vi "Write Time Remaining.vi"(8 "error in (no error)":errorcluster, 11 "Value":dbl) -> (0 "error out":errorcluster)   [LabVIEW 2015, in "UI Handler.lvclass"]
uses:
  UI Handler.lvclass
  UI Handler.lvclass/UI Handler.ctl
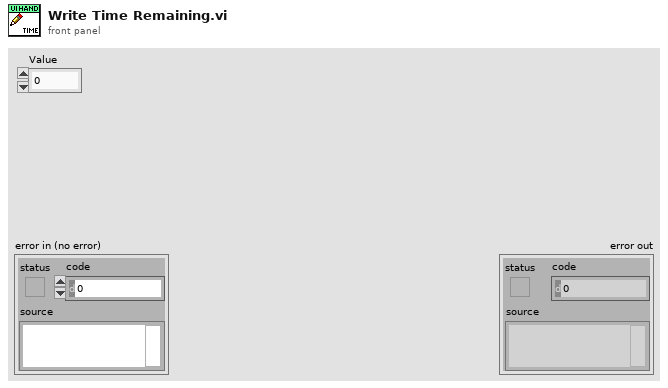
[diagram p1: front panel]
types:
  T1 = typedef "UI Handler.lvclass/Session Handle.ctl" = refnum<data-value>
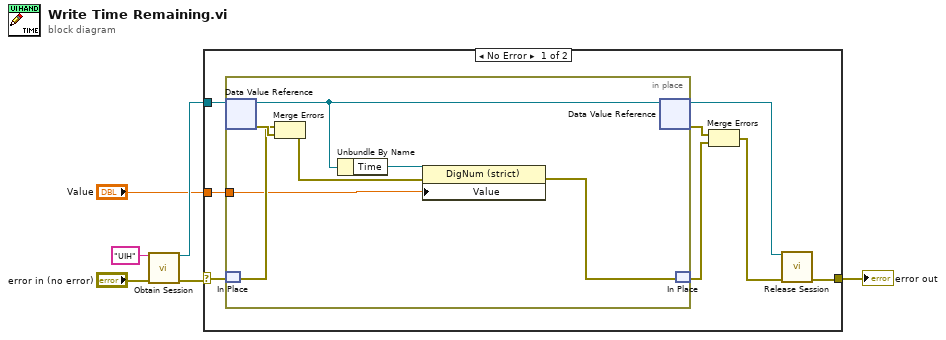
[diagram p0: block diagram]
diagram:
  n1 = call "Obtain Session.vi"("Session  Name ()"="UIH", "error in (no error)"="error in (no error)") -> ("Session Handle"=w2:T1, "error out"=w3:errorcluster)  [unwired: 12 in]
  n2 = case shown="No Error" w3 {
    selector: w3 -> [w11 w22]
    tunnel: w2 -> [w14 _]
    tunnel: [w7 w22] -> w5
    tunnel: "Value" -> [w10 _]
    frame No Error {
      n3 = in-place {
        in-place-border: w10 -> [w15]
        n4 = in-place-dvr #1(w14) -> (w19:refnum<class "UI Handler.lvclass">, w21:errorcluster)
        n5 = in-place-match #2(w11) -> (w20:errorcluster)
        n6 = Merge Errors(w20, w21) -> (w17:errorcluster)
        n7 = Unbundle By Name(w19) -> ("Time"=w18:refnum<vi>)
        n8 = property class="DigNum (strict)"(reference=w18, error in=w17, "Value"=w15) -> (error out=w16:errorcluster)  [unwired: 1 out]
        n9 = in-place-dvr #1(w19) -> (w8:T1, w12:errorcluster)
        n10 = in-place-match #2(w16) -> (w13:errorcluster)
      }
      n11 = Merge Errors(w12, w13) -> (w9:errorcluster)
      n12 = call "Release Session.vi"("Session Handle"=w8, "error in (no error)"=w9) -> ("error out"=w7:errorcluster)  [unwired: 13 in]
    }
    frame Error {
    }
  }
  "error out" <- w5
